vi "Set All Laser Powers.vi"(6 "Mode":enum16{"Normal", "Ignore", "Reset"}(ring), 7 "Correlation ID":u32, 8 "error in (no error)":errorcluster, 9 "Power":dbl, 10 "Line Enable":bool[](array[boolean]), 11 "Application in":refnum<class "Application.lvclass">) -> (0 "error out":errorcluster, 3 "Application out":refnum<class "Application.lvclass">)   [LabVIEW 2023, in "Application.lvlib" / "Application.lvclass"]
uses:
  Application.lvclass
  Application.lvclass/Application.ctl
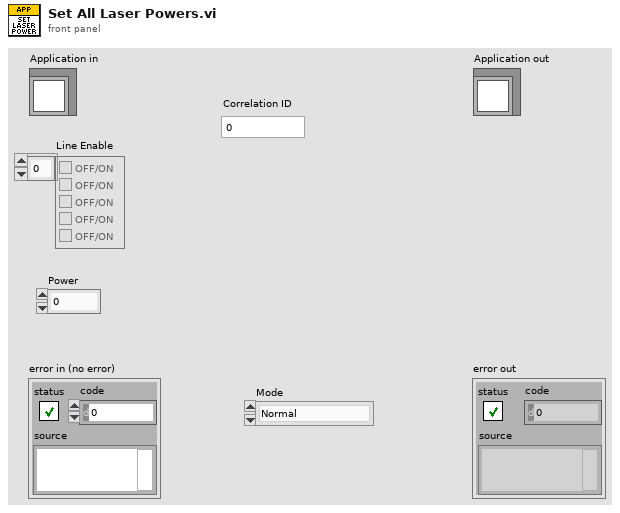
[diagram p1: front panel]
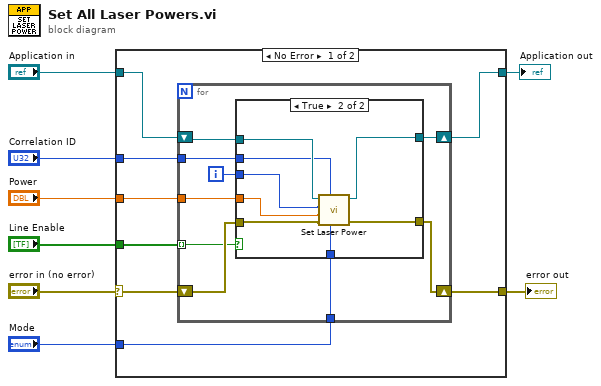
[diagram p0: block diagram]
diagram:
  n1 = case shown="No Error" "error in (no error)" {
    selector: "error in (no error)" -> [w16 w37]
    tunnel: [w15 w37] -> w7
    tunnel: [w10 w36] -> w5
    tunnel: "Application in" -> [w11 w36]
    tunnel: "Power" -> [w14 _]
    tunnel: "Mode" -> [w12 _]
    tunnel: "Line Enable" -> [w13 _]
    tunnel: "Correlation ID" -> [w9 _]
    frame No Error {
      n2 = for {
        shift-right: [w24] -> w15
        shift-left: w16 -> [w25]
        tunnel: w13 -> [w23] mode=indexing
        tunnel: w14 -> [w21]
        tunnel: w12 -> [w20]
        shift-right: [w18] -> w10
        shift-left: w11 -> [w19]
        tunnel: w9 -> [w17]
        i -> [w22]
        n3 = case shown="True" w23 {
          tunnel: w25 -> [w27 w34]
          tunnel: [w27 w35] -> w24
          tunnel: w22 -> [_ w29]
          tunnel: w21 -> [_ w30]
          tunnel: w20 -> [_ w33]
          tunnel: w19 -> [w26 w32]
          tunnel: [w26 w31] -> w18
          tunnel: w17 -> [_ w28]
          frame False {
          }
          frame True {
            n4 = call-dynamic "Set Laser Power.vi"("Mode"=w33, "Correlation ID"=w28, "error in (no error)"=w34, "Power"=w30, "laser index"=w29, "Application in"=w32) -> ("error out"=w35:errorcluster, "Application out"=w31:refnum<class "Application.lvclass">)  [unwired: 4 in]
          }
        }
      }
    }
    frame Error {
    }
  }
  "error out" <- w7
  "Application out" <- w5
